vi "CallersName.vi"(1 "Get/Set":bool, 2 "Callers Name":string) -> (0 "Callers Name out":string)   [LabVIEW 2009]
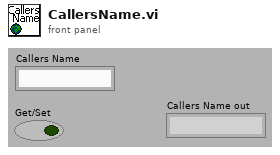
[diagram p1: front panel]
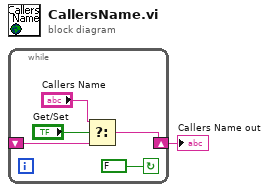
[diagram p0: block diagram]
diagram:
  n1 = while {
    shift-right: [w5] -> w1
    shift-left: _ -> [w6]
    stop <- FALSE continue-if-true
    n2 = Select(t="Callers Name", s="Get/Set", f=w6) -> (s? t:f=w5:string)
  }
  "Callers Name out" <- w1
